vi "FTW-Subscriber-RemoveAddresses.vi"(0 "FTW-Subscription In":refnum<class "FTW-Subscriber.lvclass">, 5 "Addresses":string, 11 "error in":errorcluster) -> (4 "FTW-Subscription Out":refnum<class "FTW-Subscriber.lvclass">, 15 "error out":errorcluster)   [LabVIEW 2013, in "FTW-Subscriber.lvclass"]
uses:
  FTW-Subscriber.lvclass
  FTW-Subscriber.lvclass/FTW-Subscriber.ctl
  Endpoint/FTW-Endpoint.lvclass
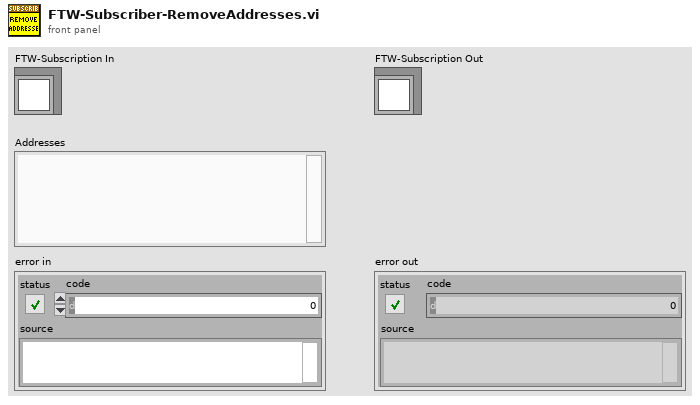
[diagram p1: front panel]
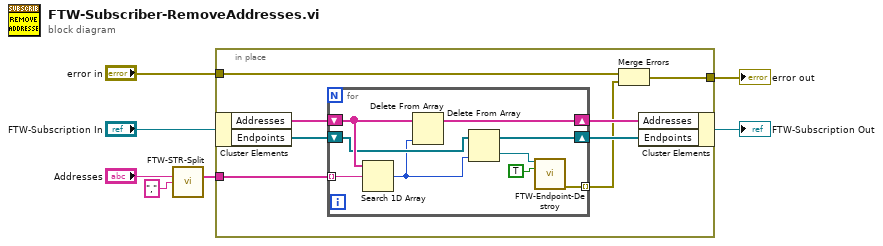
[diagram p0: block diagram]
diagram:
  n1 = call "FTW-STR-Split.vi"("Delimited String"="Addresses", "Delimiter"=",") -> ("Array of Strings"=w1:string[])  [unwired: 13 in]
  n2 = in-place {
    in-place-border: "error in" -> [w15]
    in-place-border: [w14] -> w3
    in-place-border: w1 -> [w13]
    n3 = in-place-cluster #1("FTW-Subscription In") -> ("Addresses"=w12:string[], "Endpoints"=w11:refnum<class "FTW-Endpoint.lvclass">[])
    n4 = for {
      tunnel: w13 -> [w24] mode=indexing
      shift-right: [w22] -> w10
      shift-left: w12 -> [w23]
      shift-right: [w20] -> w9
      shift-left: w11 -> [w21]
      tunnel: [w16] -> w8 mode=indexing
      n5 = Search 1D Array(1D array=w23, element=w24) -> (index of element=w19:i32)  [unwired: 1 in]
      n6 = Delete From Array(array=w23, index=w19) -> (array with subset deleted=w22:string[])  [unwired: 1 in, 1 out]
      n7 = Delete From Array(array=w21, index=w19) -> (deleted portion=w17:refnum<class "FTW-Endpoint.lvclass">, array with subset deleted=w20:refnum<class "FTW-Endpoint.lvclass">[])  [unwired: 1 in]
      n8 = call-dynamic "FTW-Endpoint-Destroy.vi"("FTW Endpoint"=w17, "Force Destroy"=TRUE ("force destroy? (F)")) -> ("error out"=w16:errorcluster)  [unwired: 13 in]
    }
    n9 = Merge Errors(w15, w8) -> (w14:errorcluster)
    n10 = in-place-cluster #1("Addresses"=w10, "Endpoints"=w9) -> (→"FTW-Subscription Out":refnum<class "FTW-Subscriber.lvclass">)
  }
  "error out" <- w3
